vi "SubVI_Example_LabVIEW_Disable_Control.vi"(11 "UI Control (Reference)":refnum<vi>) -> ()   [LabVIEW 2010]
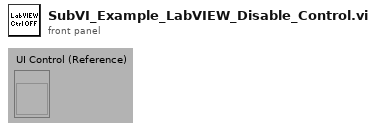
[diagram p1: front panel]
types:
  T1 = enum8{"Enabled", "Disabled", "Disabled and Grayed Out"}
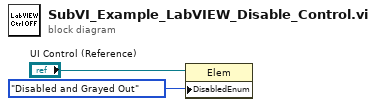
[diagram p0: block diagram]
diagram:
  n1 = property class="Elem"(reference="UI Control (Reference)", "DisabledEnum"=T1."Disabled and Grayed Out" ("Disabled")) -> ()  [unwired: 1 in, 2 out]
